vi "Set Magnet.vi"(4 "Mode":T2, 6 "Axis":T1=enum."Z", 8 "error in (no error)":errorcluster, 9 "Target Rate (T/min)":dbl, 10 "Target Field (T)":dbl, 11 "Instrument.Oxford1820 in":refnum<class "Instrument.Oxford1820.lvclass">) -> (0 "error out":errorcluster, 3 "Instrument.Oxford1820 out":refnum<class "Instrument.Oxford1820.lvclass">)   [LabVIEW 2019, in "Instrument.Oxford1820.lvclass"]
uses:
  Instrument.Oxford1820.lvclass
  C:/Program Files (x86)/National Instruments/LabVIEW 2019/user.lib/LevyLab/Instrument Framework/Instrument/Instrument.lvclass
  <userlib>/LevyLab/Instrument Framework/Instrument Types/Cryostat/Typedefs/Magnet Mode--Enum.ctl
  <userlib>/LevyLab/Instrument Framework/Instrument Types/Cryostat/Typedefs/Magnet Axis--Enum.ctl
  Typedefs/Instrument.Oxford1820.Commands-enum.ctl
  <userlib>/LevyLab/Instrument Framework/Instrument Types/Cryostat/Typedefs/setMagnet--cluster.ctl
  d8f78421-19f3-442f-b366-e122dd2883f1.vi
  d8f78421-19f3-442f-b366-e122dd2883f1.vi/1850c8cd-d171-4f21-82b9-a7b75d686c1d.vi
  d8f78421-19f3-442f-b366-e122dd2883f1.vi/1850c8cd-d171-4f21-82b9-a7b75d686c1d.vi/374dd196-eca9-4076-b307-184e6bb6b47a.vi
  d8f78421-19f3-442f-b366-e122dd2883f1.vi/1850c8cd-d171-4f21-82b9-a7b75d686c1d.vi/76e09a6c-2f31-4200-ad45-086c1a27d77a.vi
  <userlib>/LevyLab/Instrument Framework/Instrument/API/RemoteClient.vi
  <vilib>/Utility/Data Type/Get Type Information.vi
  <vilib>/JDP Science/JSONtext/JSON text to Variant.vi
  <vilib>/JDP Science/JSONtext/LVClass Serializer/JSONtext LVClass Serializer.lvclass
  <userlib>/LevyLab/Instrument Framework/Instrument Types/Cryostat/Instrument.Cryostat.lvclass
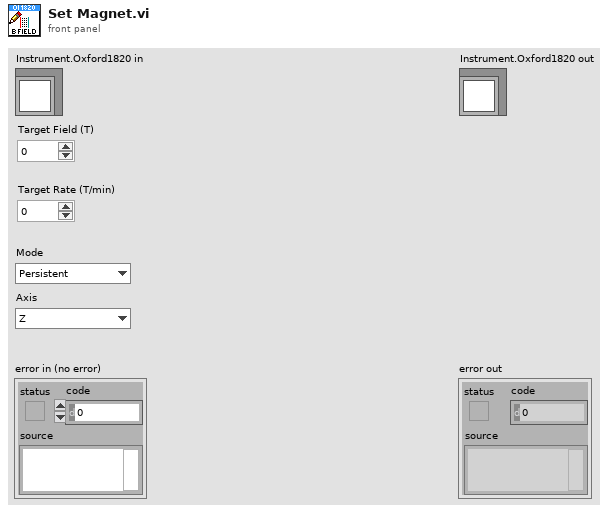
[diagram p1: front panel]
types:
  T1 = typedef "Instrument.Cryostat.lvclass/Magnet Axis--Enum.ctl" = enum16{"X", "Y", "Z"}
  T2 = typedef "Instrument.Cryostat.lvclass/Magnet Mode--Enum.ctl" = enum16{"Persistent", "Driven"}
  T3 = typedef "Instrument.Cryostat.lvclass/setMagnet--cluster.ctl" = cluster{"field":dbl, "rate":dbl, "axis":T1, "mode":T2}
  T4 = typedef "Instrument.Oxford1820.lvclass/Instrument.Oxford1820.Commands-enum.ctl" = enum16{"setAction", "setTarget", "setSwitchHeat", "setLambda", "setFillMode", "setNeedleValve", "setMagnetField", "getStatus", "getTarget", "getSwitchHeat", "getPSUField", "setSequenceStatus", "getMagnetField"}
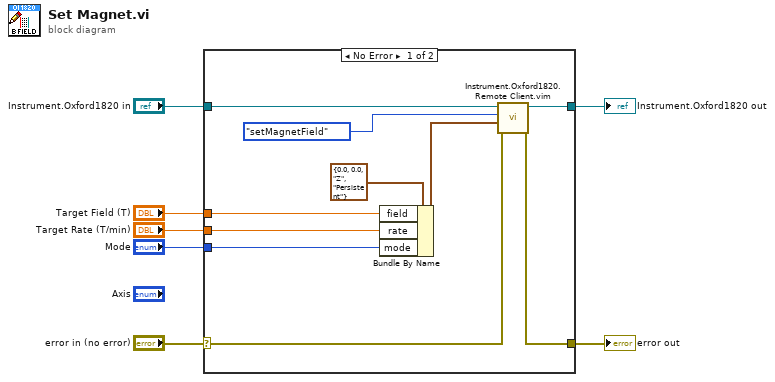
[diagram p0: block diagram]
diagram:
  n1 = case shown="No Error" "error in (no error)" {
    selector: "error in (no error)" -> [w14 w19]
    tunnel: "Mode" -> [w9 _]
    tunnel: "Target Rate (T/min)" -> [w8 _]
    tunnel: [w13 w19] -> w5
    tunnel: "Target Field (T)" -> [w17 _]
    tunnel: "Instrument.Oxford1820 in" -> [w16 w18]
    tunnel: [w15 w18] -> w1
    frame No Error {
      n2 = Bundle By Name(cluster=T3 {"field"=0.0, "rate"=0.0, "axis"=enum."Z", "mode"=enum."Persistent"} ("Set Magnet Field"), "field"=w17, "rate"=w8, "mode"=w9) -> (w12:T3)
      n3 = call "Instrument.Oxford1820.Remote Client.vim"("error in (no error)"=w14, "Data"=w12, "Commands"=Instrument.Oxford1820.Commands-enum."setMagnetField", "Instrument.1820 in"=w16) -> ("error out"=w13:errorcluster, "Instrument.1820 out"=w15:refnum<class "Instrument.Oxford1820.lvclass">)  [unwired: 5 in, 1 out]
    }
    frame Error {
    }
  }
  "Instrument.Oxford1820 out" <- w1
  "error out" <- w5
